vi "校准记录读取.vi"(1 "测量参数":u16(ring) items=["COD"=22, "氨氮"=3, "总氮"=2, "总磷"=1], 2 "测量模式":T1(ring), 3 "量程":enum16{"低量程", "高量程"}(ring), 11 "Error in":errorcluster caption="Error in (no error)") -> (4 "MB session out":refnum<class "MB_Master.lvclass">, 6 "校准记录":T2, 15 "error out":errorcluster)   [LabVIEW 2016, in "斯坦道总磷.lvlib"]
uses:
  <vilib>/Plasmionique/MB Master/MB_Master/MB_Master.lvclass
  <vilib>/Plasmionique/MB Master/MB Master.lvlib
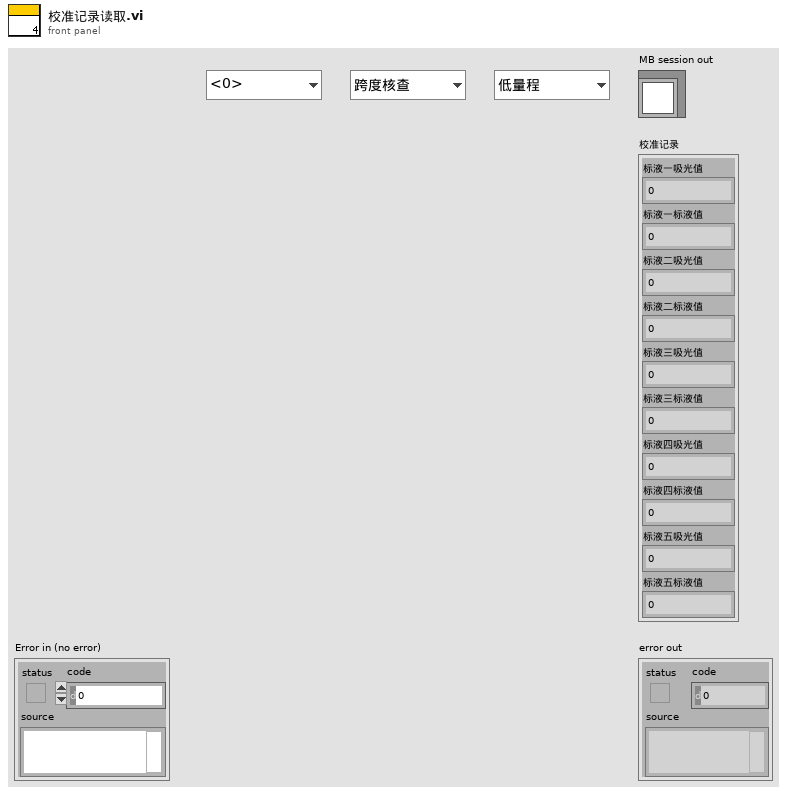
[diagram p1: front panel]
types:
  T1 = enum16{"跨度核查", "水样测量", "零点核查", "标样核查", "加标回收", "快捷测试", "空白校准", "标样校准"}
  T2 = cluster{"标液一吸光值":sgl, "标液一标液值":sgl, "标液二吸光值":sgl, "标液二标液值":sgl, "标液三吸光值":sgl, "标液三标液值":sgl, "标液四吸光值":sgl, "标液四标液值":sgl, "标液五吸光值":sgl, "标液五标液值":sgl}
  T3 = cluster{"FLOAT[0]":sgl, "FLOAT[1]":sgl, "FLOAT[2]":sgl, "FLOAT[3]":sgl, "FLOAT[4]":sgl, "FLOAT[5]":sgl, "FLOAT[6]":sgl, "FLOAT[7]":sgl, "FLOAT[8]":sgl, "FLOAT[9]":sgl}
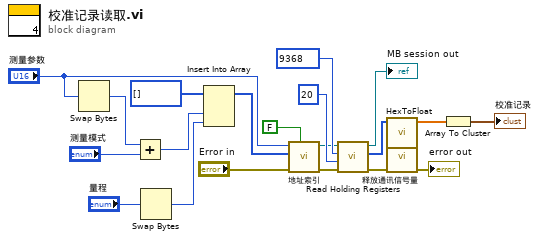
[diagram p0: block diagram]
diagram:
  n1 = Swap Bytes(anything="测量参数") -> (byte swapped=w12:u16)
  n2 = Add(x=w12, y="测量模式") -> (x+y=w14:u16)
  n3 = Swap Bytes(anything="量程") -> (byte swapped=w11:u16)
  n4 = Insert Into Array(array=u16[] [] ("数组"), new element #1=w14, new element #2=w11) -> (w7:u16[])  [unwired: 1 in]
  n5 = call "地址索引.vi"("4.2写公式？"=FALSE, "error in (no error)"="Error in", "values"=w7, "测量参数"="测量参数") -> ("error out"=w4:errorcluster, "MB session out"=w5:refnum<class "MB_Master.lvclass">)  [unwired: 6 in]
  n6 = call <vilib>:"Read Holding Registers.vi"("error in (no error)"=w4, "quantity"=u16 20, "starting address"=u16 9368, "MB session in"=w5) -> ("error out"=w3:errorcluster, "Registers"=w16:u16[], "MB session out"=→"MB session out":refnum<class "MB_Master.lvclass">)  [unwired: 5 in]
  n7 = call "HexToFloat.vi"("数组"=w16) -> ("FLOAT"=w15:sgl[])  [unwired: 10 in]
  n8 = call "释放通讯信号量.vi"("error in (no error)"=w3) -> ("error out"=→"error out":errorcluster)  [unwired: 10 in]
  n9 = Array To Cluster(array=w15) -> (cluster=→"校准记录":T3)
